vi "FFT_lookuptable_sum.vi"() -> ()   [LabVIEW 2020]
uses:
  <vilib>/rvi/DataTransferAndStorage/Container/XNode/niFpgaContainer.xnode
  <vilib>/rvi/interface/RandomDataEmulation/nirviRandomDataFpgaReadWriteTemplate.vi
  <vilib>/rvi/FIFO/Fifo_Resource/niFpgaFifoEmulationRefIn.vi
  <vilib>/fxp/LVFixedPointQuantizationPolicyTypeDef.ctl
  <vilib>/rvi/Analysis/measure/FFT/simModelSupport/niFpgaFFTSimDfxp.ctl
  <vilib>/rvi/Analysis/measure/FFT/simModelSupport/niFpgaFFTSimArithmeticProperties.ctl
  <vilib>/rvi/Analysis/measure/FFT/simModelSupport/niFPGA FFT Sim Types.ctl
  <vilib>/rvi/Analysis/measure/FFT/simModelSupport/niFPGA FFT Outside SCTL Sim Properties.ctl
  <vilib>/rvi/Analysis/measure/FFT/simModelSupport/niFpgaFFTSimModelOutsideSCTLCore.vi
  <vilib>/rvi/Analysis/measure/FFT/XNode/niFpgaFFT.xnode
  <vilib>/rvi/FXPMathLib/FxpSinAndCos/subVIs/nifxpmath_SinAndCos_SimConfig.ctl
  <vilib>/rvi/FXPMathLib/FxpSinAndCos/simVIs/DllFxpSinAndCosTemp_sub.vi
  <vilib>/rvi/FXPMathLib/FxpSinAndCos/XNode/nifxpmath_SinAndCos.xnode
  <vilib>/rvi/LocalResourceManager/LocalResourceManager.xnode
  <vilib>/rvi/eio/common/nirviEmuReportErrorAndStop.vi
  <vilib>/rvi/DataTransferAndStorage/Container/Common/niFpgaContainerGetUniqueNameForEmu.vi
  <vilib>/rvi/DataTransferAndStorage/Container/Common/niFpgaContainerSetEmuInfo.vi
panel:
  out "x+y":fxp<+/-,33,17>[](array[numeric])
  out "Numeric 3":i32
  out "val":fxp<+,64,48>
  out "n*d":fxp<+,32,16>
  out "size(s)":i32
  out "N":fxp<+/-,18,17>
  in  "n":fxp<+,32,16>
  in  "s (sample rate)":fxp<+,32,16>
  out "Numeric":i32
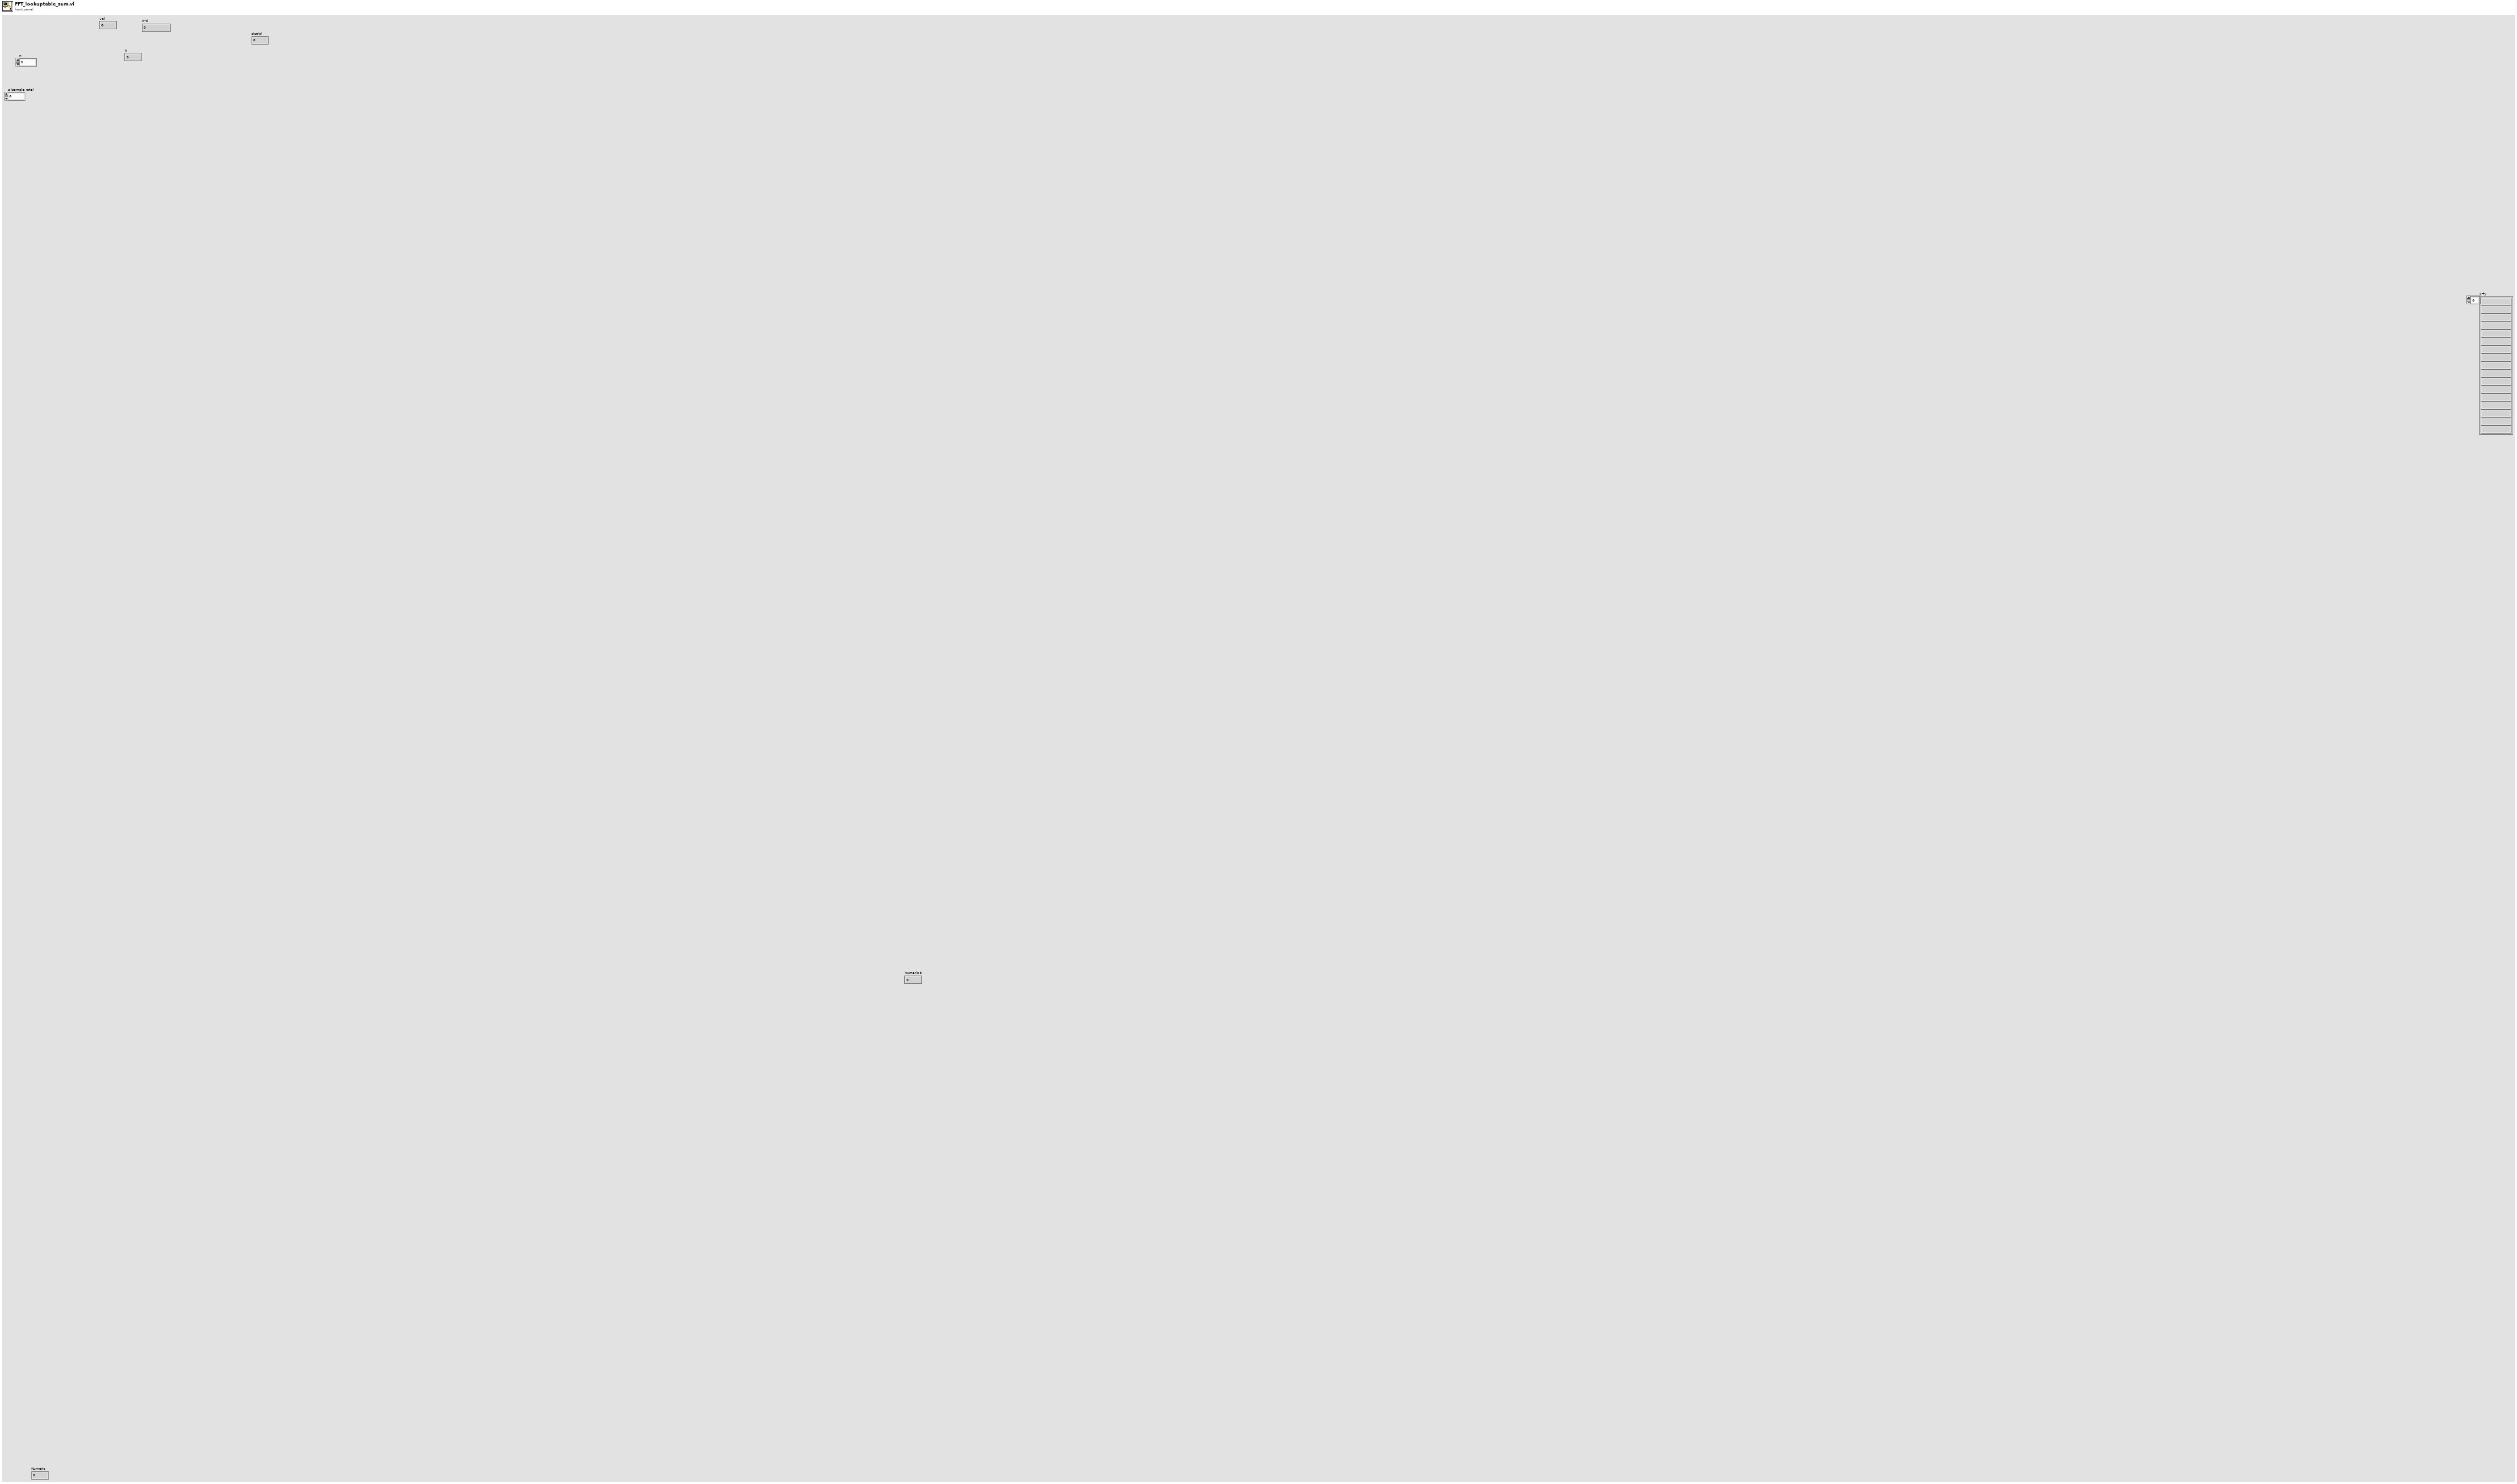
[diagram p1: front panel]
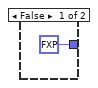
[diagram p2: hidden frame]
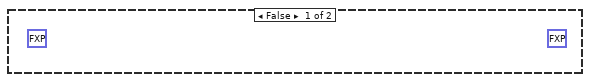
[diagram p3: hidden frame]
diagram:
  (unwired) fxp<+/-,32,16> 0.0
  w3 = 512  # sample rate/input
  w2 = 128  # FFT size
  # "restored_sig += ampli * np.cos(2 * np.pi * (f[j]*Ts * t1 + phase))"
  # ">> frequency interval (delta)>>"
  # "https://www.edn.com/tip-ffts-in-labview-fpga/"
  n1 = xnode "VI-Defined FIFO Configuration"() -> ("FIFO Out"=w12:refnum<k21>)
  n2 = flat-sequence {
    tunnel: w12 -> [w15]
    tunnel: w12 -> [w23]
    tunnel: w11 -> [w22]
    tunnel: w10 -> [w21]
    tunnel: w11 -> [w204]
    tunnel: w10 -> [w203]
    tunnel: w9 -> [w202]
    tunnel: w8 -> [w201]
    tunnel: [w200] -> w13
    tunnel: w9 -> [w238]
    tunnel: w8 -> [w237]
    tunnel: w13 -> [_]
    frame #0 {
      # "data input from host to target"
      n3 = for {
        N: 766 -> [_]
        tunnel: w15 -> [w19]
        i -> [w16]
        n4 = xnode ("FIFO Read")("Timeout"=0) -> ("Element"=w17:fxp<+/-,24,7>)  [unwired: 1 in, 2 out]
        n5 = xnode ("FIFO Write")("Element"=w17, "Timeout"=0, "FIFO In"=w19) -> ()  [unwired: 2 out]
        "Numeric" <- w16
      }
    }
    frame #1 {
      # "FFT based prediction whole process"
      n6 = while {
        tunnel: w23 -> [w33]
        tunnel: w22 -> [w26]
        tunnel: w21 -> [w25]
        tunnel: [w24] -> _
        i -> [w32]
        stop <- w27 stop-if-true
        n7 = flat-sequence {
          tunnel: w33 -> [w37]
          tunnel: [w36] -> w31
          tunnel: [w35] -> w24
          tunnel: w31 -> [w47]
          tunnel: [w46] -> w30
          tunnel: [w45] -> w29
          tunnel: [w44] -> w28
          tunnel: w30 -> [w72]
          tunnel: w29 -> [w71]
          tunnel: w28 -> [w68]
          tunnel: w26 -> [w70]
          tunnel: w25 -> [w69]
          frame #0 {
            w35 = TRUE
            # "signal input through FIFO iteam"
            n8 = case shown="True" w35 {
              tunnel: w37 -> [_ w41]
              tunnel: [fxp<+/-,24,7> 0.0 ("Element") w39] -> w36
              frame False {
              }
              frame True {
                n9 = xnode ("FIFO Write")("Timeout"=0, "FIFO In"=w41) -> ("Element"=w39:fxp<+/-,24,7>)  [unwired: 2 out]
              }
            }
          }
          frame #1 {
            # "FFT function for getting real and imaginary values"
            n10 = xnode ("FIFO Write")("Element"=w47, "Timeout"=0) -> ()  [unwired: 1 in, 2 out]
            n11 = xnode ("FFT")("real data in"=w47, "reset"=FALSE) -> ("real data out"=w46:fxp<+/-,32,15>, "imaginary data out"=w45:fxp<+/-,32,15>, "output valid"=w44:bool)  [unwired: 1 in, 1 out]
          }
          frame #2 {
            # "measuring magnitude, phase and frequencies"
            n12 = case shown="True" w68 {
              tunnel: w71 -> [_ w88]
              tunnel: w72 -> [_ w87]
              tunnel: w70 -> [_ w77]
              tunnel: w69 -> [_ w73]
              frame False {
                (unwired) fxp<+/-,32,16> 0.0
                (unwired) fxp<+/-,32,16> 0.0
              }
              frame True {
                # "magnitude=root (x^2+y^2)\nwhere, x=real and y=imag"
                # "phase=arctan(img(Y)/real(x))\nhere in FPGA we don't have arctan\nso m odified arctan=cos/sine\nphase=cos(z)/sine(z), where z=(y/x)"
                n13 = Square(x=w87) -> (x^2=w82:fxp<+,63,29>)
                n14 = Square(x=w88) -> (x^2=w76:fxp<+,63,29>)
                n15 = Divide(x=w88, y=w87) -> (x/y=w80:fxp<+/-,32,16>)
                n16 = xnode "High Throughput Sine & Cosine"("x (pi)"=w80) -> ("sin(x)"=w83:fxp<+/-,32,2>, "cos(x)"=w84:fxp<+/-,32,2>)
                n17 = Divide(x=w84, y=w83) -> (x/y=w75:fxp<+/-,32,16>)
                n18 = xnode ("FIFO Write")("Element"=w75, "Timeout"=0) -> ()  [unwired: 1 in, 2 out]
                n19 = xnode ("FIFO Write")("Element"=w75, "Timeout"=0, "FIFO In"=w73) -> ()  [unwired: 2 out]
                n20 = Add(x=w82, y=w76) -> (x+y=w81:fxp<+,64,30>)
                n21 = Square Root(x=w81) -> (sqrt(x)=w79:fxp<+/-,32,16>)
                n22 = xnode ("FIFO Write")("Element"=w79, "Timeout"=0) -> ()  [unwired: 1 in, 2 out]
                n23 = xnode ("FIFO Write")("Element"=w79, "Timeout"=0, "FIFO In"=w77) -> ()  [unwired: 2 out]
              }
            }
          }
        }
        n24 = Greater?(x=w32, y=766 ("Timeout")) -> (0:w27:bool)
      }
    }
    frame #2 {
    }
    frame #3 {
      n25 = flat-sequence {
        tunnel: ["n"] -> w138
        tunnel: ["s (sample rate)"] -> _
        tunnel: ["n"] -> _
        tunnel: ["s (sample rate)"] -> w137
        tunnel: ["n"] -> w136
        tunnel: ["n"] -> w135
        tunnel: [w145] -> w134
        tunnel: w138 -> [w144]
        tunnel: w137 -> [w143]
        tunnel: [w143] -> w133
        tunnel: w136 -> [w142]
        tunnel: [w142] -> w132
        tunnel: w135 -> [w141]
        tunnel: [w141] -> w131
        tunnel: w134 -> [w157]
        tunnel: [w155] -> w130
        tunnel: w133 -> [w154]
        tunnel: [w154] -> w129
        tunnel: w132 -> [w153]
        tunnel: [w153] -> w128
        tunnel: w131 -> [w152]
        tunnel: [w152] -> w127
        tunnel: [w168] -> w126
        tunnel: [w164] -> _
        tunnel: w130 -> [w164]
        tunnel: w129 -> [w167]
        tunnel: [w167] -> w125
        tunnel: w128 -> [w166]
        tunnel: w127 -> [w165]
        tunnel: [w165] -> w124
        tunnel: [w164] -> w123
        tunnel: w126 -> [w184]
        tunnel: w125 -> [w183]
        tunnel: [w183] -> w122
        tunnel: [w182] -> w121
        tunnel: [w182] -> w120
        tunnel: w124 -> [w181]
        tunnel: [w181] -> w119
        tunnel: w123 -> [w180]
        tunnel: w122 -> [w190]
        tunnel: w121 -> [w189]
        tunnel: w120 -> [w188]
        tunnel: w119 -> [w187]
        frame #0 {
          # "n=windowlength\ns= sample rate\nd=inverserse of sampling rate in numpy\ns=1/d"
        }
        frame #1 {
          # "N=(n-1)//2+1"
          n26 = Subtract(x=w144, y=fxp<+,1,1> 1.0) -> (x-y=w149:fxp<+/-,33,17>)
          n27 = Divide(x=w149, y=fxp<+,1,2> 2.0) -> (x/y=w150:fxp<+/-,34,16>)
          n28 = Round Toward -Infinity(1:w150) -> (0:w151:fxp<+/-,16,16>)
          n29 = Add(x=w151, y=fxp<+,1,1> 1.0) -> (x+y=w145:fxp<+/-,18,17>)
          "N" <- w145
        }
        frame #2 {
          # "p1=arange(0,N,dtype=int)"
          n30 = To Long Integer(number=w157) -> (32bit integer=w158:i32)
          n31 = for {
            N: w158 -> [_]
            shift-right: [w159] -> _
            shift-left: fxp<+,1,1> 0.0 -> [w161]
            shift-right: [w162] -> w155
            shift-left: _ -> [w163]
            n32 = Increment(x=w161) -> (x+1=w160:fxp<+/-,33,33>)
            n33 = Build Array (concatenate)(w163, w161) -> (w162:fxp<+/-,32,32>[])
            n34 = To Long Integer(number=w160) -> (32bit integer=w159:i32)
          }
        }
        frame #3 {
          # "p2 =arange(-(n//2),0,dtype=int)"
          n35 = Divide(x=w166, y=fxp<+,1,2> 2.0) -> (x/y=w171:fxp<+,33,15>)
          n36 = Round Toward -Infinity(1:w171) -> (0:w173:fxp<+,15,15>)
          n37 = To Long Integer(number=w173) -> (32bit integer=w172:i32)
          n38 = for {
            N: w172 -> [_]
            shift-right: [w175] -> _
            shift-left: fxp<+,1,1> 0.0 -> [w177]
            shift-right: [w178] -> w174
            shift-left: _ -> [w179]
            n39 = Decrement(x=w177) -> (x-1=w176:fxp<+/-,33,33>)
            n40 = Build Array (concatenate)(w179, w177) -> (w178:fxp<+/-,32,32>[])
            n41 = To Long Integer(number=w176) -> (32bit integer=w175:i32)
          }
          n42 = Reverse 1D Array(array=w174) -> (reversed array=w168:fxp<+/-,32,32>[])
        }
        frame #4 {
          # "results=empty(n,int)\nresults[:N]=p1\nresults[N:]=p2"
          n43 = Insert Into Array(array=w180, new element=w184) -> (w182:fxp<+/-,32,32>[])  [unwired: 1 in]
        }
        frame #5 {
          # "val=1/(n*d)\nf=results*val"
          n44 = Divide(x=w187, y=w190) -> (x/y=w193:fxp<+,64,32>)
          "n*d" <- w193
          n45 = Array Size(array=w189) -> (size(s)=w192:i32)
          n46 = Divide(x=fxp<+,32,32> 1.0, y=w193) -> (x/y=w194:fxp<+,32,16>)
          "val" <- w194
          n47 = Round Toward -Infinity(1:w194) -> (0:w195:fxp<+,16,16>)
          n48 = for {
            N: w192 -> [_]
            tunnel: w195 -> [w199]
            tunnel: [w197] -> w186 mode=indexing
            tunnel: w188 -> [w198] mode=indexing
            n49 = Multiply(x=w198, y=w199) -> (x*y=w197:fxp<+/-,32,16>)
            n50 = xnode ("FIFO Write")("Element"=w197, "Timeout"=0) -> ()  [unwired: 1 in, 2 out]
          }
          n51 = Array Size(array=w186) -> (size(s)=→"size(s)":i32)
        }
      }
    }
    frame #4 {
      w200 = fxp<+/-,32,16>[] [128.0, 132.0, 136.0, 252.0, 256.0, 260.0, 380.0, 384.0, 388.0, -128.0, -132.0, -136.0, -252.0, -256.0, -260.0, -380.0, -384.0, -388.0]  # selective frequencies
      w209 = 512  # sample rate/input
      w210 = 128  # FFT size
      # "GOAL:\n1. build a list of frequencies\n2. use the list for building a forloop"
      # "What done?\n1. make a array of 18 frequencies\n2. devide frequency array with frequency interval(delta) to get its sample points\n3. to get specific magnitude and phase of the specific frequency use index array through a for loop\n5. get magnitude and phase of that 28 frequencies."
      # ">> frequency interval (delta)>>"
      # "collect specific frequencies"
      n52 = for {
        N: 512 -> [_]
        tunnel: [w230] -> w208 mode=indexing
        tunnel: [w229] -> w207 mode=indexing
        tunnel: w204 -> [w228]
        tunnel: w203 -> [w227]
        n53 = xnode ("FIFO Write")("Timeout"=0, "FIFO In"=w228) -> ("Element"=w229:fxp<+/-,32,16>)  [unwired: 2 out]
        n54 = xnode ("FIFO Write")("Timeout"=0, "FIFO In"=w227) -> ("Element"=w230:fxp<+/-,32,16>)  [unwired: 2 out]
      }
      n55 = To Fixed-Point(number=w209) -> (fixed-point=w212:fxp<+/-,32,32>)  [unwired: 1 in]
      n56 = To Fixed-Point(number=w210) -> (fixed-point=w211:fxp<+/-,32,32>)  [unwired: 1 in]
      n57 = Divide(x=w212, y=w211) -> (x/y=w213:fxp<+/-,32,16>)
      n58 = Divide(x=w200, y=w213) -> (x/y=w214:fxp<+/-,32,16>[])
      n59 = To Long Integer(number=w214) -> (32bit integer=w206:i32[])
      n60 = for {
        tunnel: w206 -> [w225] mode=indexing
        tunnel: w208 -> [w224]
        tunnel: w207 -> [w223]
        tunnel: w202 -> [w220]
        tunnel: w201 -> [w215]
        i -> [w226]
        n61 = Index Array(array=w223, index=w225) -> (element=w217:fxp<+/-,32,16>)
        n62 = Index Array(array=w224, index=w225) -> (element=w219:fxp<+/-,32,16>)
        n63 = xnode ("FIFO Write")("Element"=w217, "Timeout"=0, "FIFO In"=w215) -> ()  [unwired: 2 out]
        n64 = xnode ("FIFO Write")("Element"=w217, "Timeout"=0) -> ()  [unwired: 1 in, 2 out]
        n65 = xnode ("FIFO Write")("Element"=w219, "Timeout"=0) -> ()  [unwired: 1 in, 2 out]
        n66 = xnode ("FIFO Write")("Element"=w219, "Timeout"=0, "FIFO In"=w220) -> ()  [unwired: 2 out]
        "Numeric 3" <- w226
      }
    }
    frame #5 {
      (unwired) fxp<+/-,32,16>[] [1.0, 2.0, 3.0, 4.0, 5.0, 6.0]  # array list
      # "1. build extended time(t1)\n2. use restored signal equation to get each signal of each frequency\n3. use a transpose 2D array > forloop to sum all frequencies and get restored signal."
      # "extended time"
      n67 = for {
        N: 18 -> [_]
        tunnel: w238 -> [w244]
        tunnel: w237 -> [w246]
        tunnel: [w242] -> w235 mode=indexing
        tunnel: [w241] -> w234 mode=indexing
        n68 = xnode ("FIFO Write")("Timeout"=0, "FIFO In"=w246) -> ("Element"=w241:fxp<+/-,32,16>)  [unwired: 2 out]
        n69 = xnode ("FIFO Write")("Timeout"=0, "FIFO In"=w244) -> ("Element"=w242:fxp<+/-,32,16>)  [unwired: 2 out]
      }
      n70 = Add(x=w235, y=w234) -> (x+y=w233:fxp<+/-,33,17>[])
      "x+y" <- w233
      n71 = for {
        tunnel: w233 -> [w240] mode=indexing
        n72 = xnode ("FIFO Write")("Element"=w240, "Timeout"=0) -> ()  [unwired: 1 in, 2 out]
      }
      n73 = Multiply() -> ()  [unwired: 2 in, 1 out]
    }
  }
  n74 = xnode "VI-Defined FIFO Configuration"() -> ("FIFO Out"=w11:refnum<k21>)
  n75 = xnode "VI-Defined FIFO Configuration"() -> ("FIFO Out"=w10:refnum<k21>)
  n76 = xnode "VI-Defined FIFO Configuration"() -> ("FIFO Out"=w8:refnum<k21>)
  n77 = xnode "VI-Defined FIFO Configuration"() -> ("FIFO Out"=w9:refnum<k21>)
  n78 = To Fixed-Point(number=w3) -> (fixed-point=w6:fxp<+/-,32,32>)  [unwired: 1 in]
  n79 = To Fixed-Point(number=w2) -> (fixed-point=w7:fxp<+/-,32,32>)  [unwired: 1 in]
  n80 = Divide(x=w6, y=w7) -> (x/y=w4:fxp<+/-,32,16>)
  n81 = feedback #1() -> (w5:fxp<+/-,32,16>)  [unwired: 1 in]
  n82 = Add(x=w5, y=w4) -> (x+y=w1:fxp<+/-,32,16>)
  n83 = feedback-in #1(w1) -> ()
